vi "FVIR_LDO_Alicat_GasMeter.vi"(8 "error in":errorcluster, 11 "Message Queues":T1) -> (0 "error out":errorcluster)   [LabVIEW 2020]
uses:
  Message Queue/All Message Queues.ctl
  Message Queue/Message Cluster.ctl
  Modbus/Modbus Gas Meter Data.ctl
  Drivers/Alicat LabVIEW Drivers 2v1/Sub-VIs/Data Cluster.ctl
  Drivers/Alicat LabVIEW Drivers 2v1/Sub-VIs/Units of Measure.ctl
  Message Queue/Enqueue Message (Single).vi
  Message Queue/Message Queue.lvlib
panel:
  out "Numeric":i32
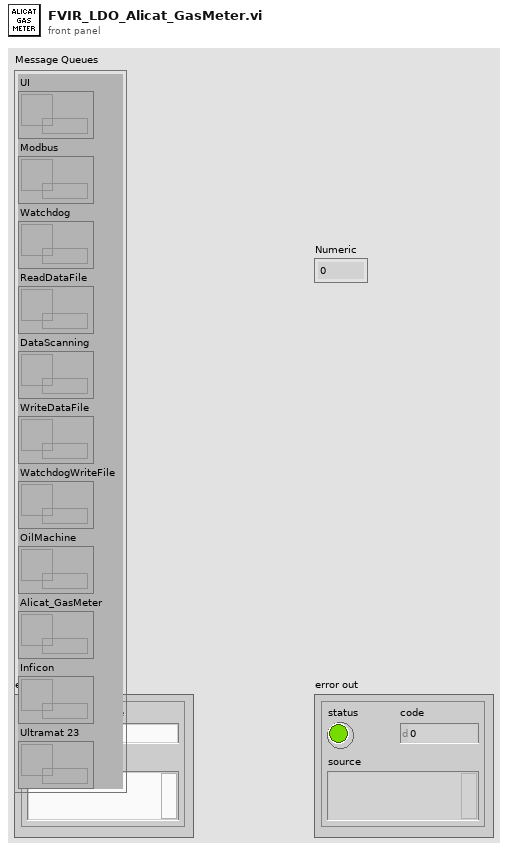
[diagram p1: front panel]
types:
  T1 = typedef "Message Queue.lvlib/All Message Queues.ctl" = cluster{"UI":refnum<queue>, "Modbus":refnum<queue>, "Watchdog":refnum<queue>, "ReadDataFile":refnum<queue>, "DataScanning":refnum<queue>, "WriteDataFile":refnum<queue>, "WatchdogWriteFile":refnum<queue>, "OilMachine":refnum<queue>, "Alicat_GasMeter":refnum<queue>, "Inficon":refnum<queue>, "Ultramat 23":refnum<queue>}
  T2 = cluster{"Absolute Press.":bool, "Gauge/Diff. Press.":bool, "Barometric Press.":bool, "Temperature":bool, "Volumetric":bool, "Mass Flow":bool, "Setpoint":bool, "Valve Drive":bool, "Totalizer":bool, "Tot. Timer [s]":bool, "Tot. Avg. Flow":bool, "Tot. Peak Flow":bool, "Gas Selected":bool, "Log Data":bool}
  T3 = typedef "Modbus Gas Meter Data.ctl" = cluster{"Data Cluster":T4, "Units of Measure Input":T5, "Header Array":string[]}
  T4 = typedef "Data Cluster.ctl" = cluster{"Absolute Pressure":dbl, "Gauge/Diff. Pressure":dbl, "Barometric Pressure":dbl, "Temperature":dbl, "Volumetric Flow":dbl, "Mass Flow":dbl, "Setpoint":dbl, "Valve Drive":dbl, "Totalizer":dbl, "[hr]":dbl, "[min]":dbl, "[sec]":dbl, "Totalizer Average Flow":dbl, "Totalizer Peak Flow":dbl, "Gas selected":string}
  T5 = typedef "Units of Measure.ctl" = cluster{"Abs. Pressure":string, "Gauge/Diff. Press.":string, "Barometric Press.":string, "Temperature":string, "Volume":string, "Mass":string, "Setpoint":string, "Valve Drive":string, "Totalizer":string, "Tot. Timer":string, "Tot. Avg. Flow":string, "Tot. Peak Flow":string}
  T6 = typedef "Data Frame.ctl" = cluster{"Absolute Pressure":bool, "Gauge/Diff. Pressure":bool, "Barometric Pressure":bool, "Temperature":bool, "Volumetric":bool, "Mass":bool, "Setpoint":bool, "Valve Drive":bool, "Totalizer":bool, "Totalizer Timer":bool, "Totalizer Average Flow":bool, "Totalizer Peak Flow":bool, "Gas Selected":bool, "Tot. Timer Format":u16}
  T7 = typedef "FMA1600A Units String.ctl" = cluster{"Software Rev":string, "Model Number":string, "Manufacturer Info":string, "Software Sub-Rev":string, "Board Rev":string, "Units of Measure Input":T5}
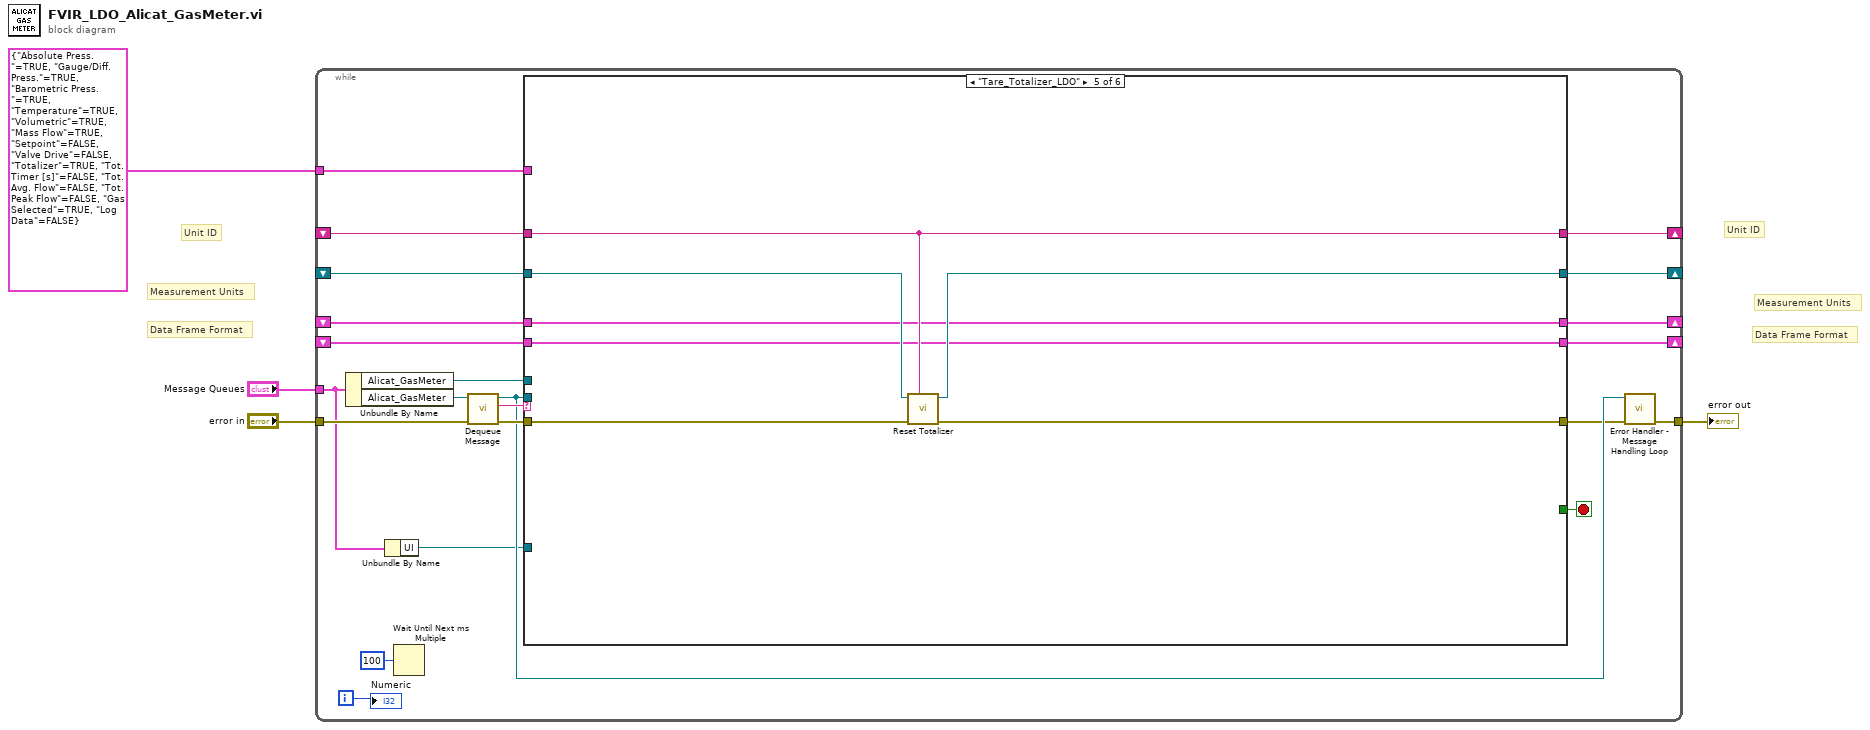
[diagram p0: block diagram]
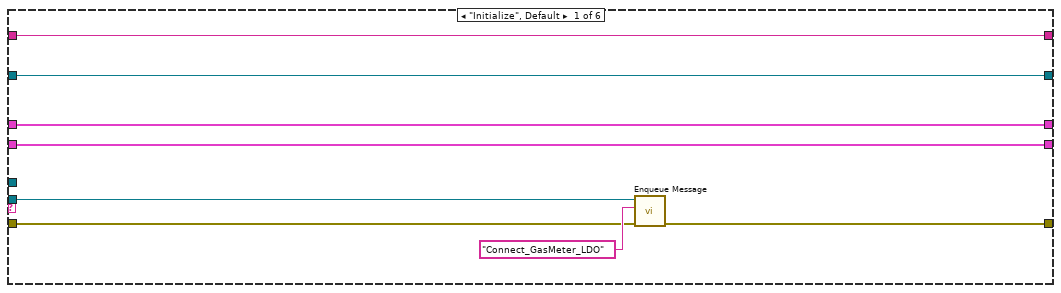
[diagram p2: hidden frame]
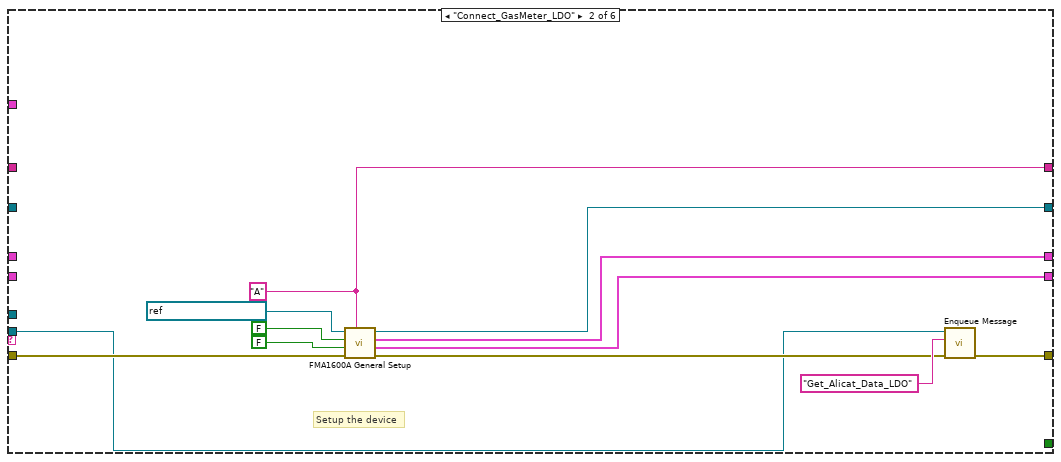
[diagram p3: hidden frame]
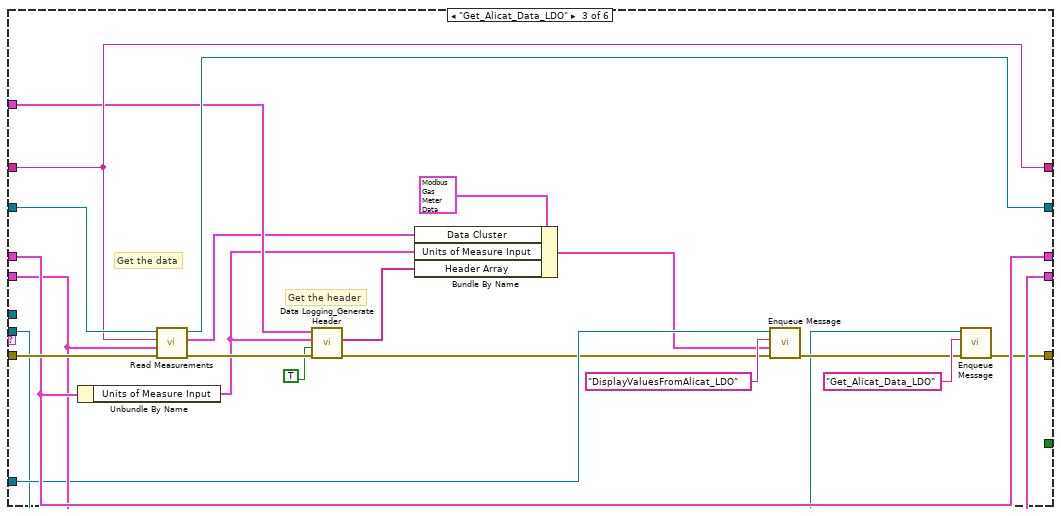
[diagram p4: hidden frame]
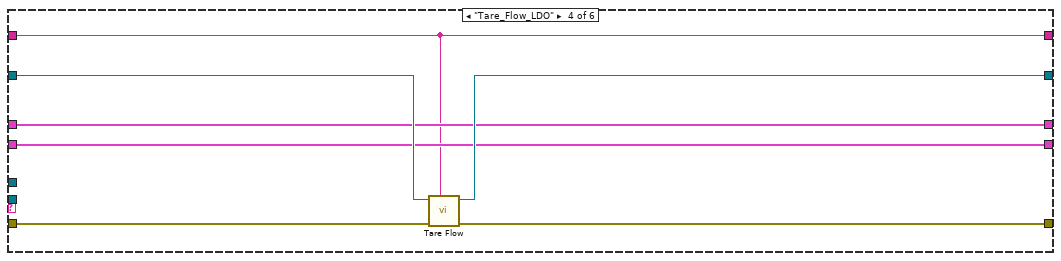
[diagram p5: hidden frame]
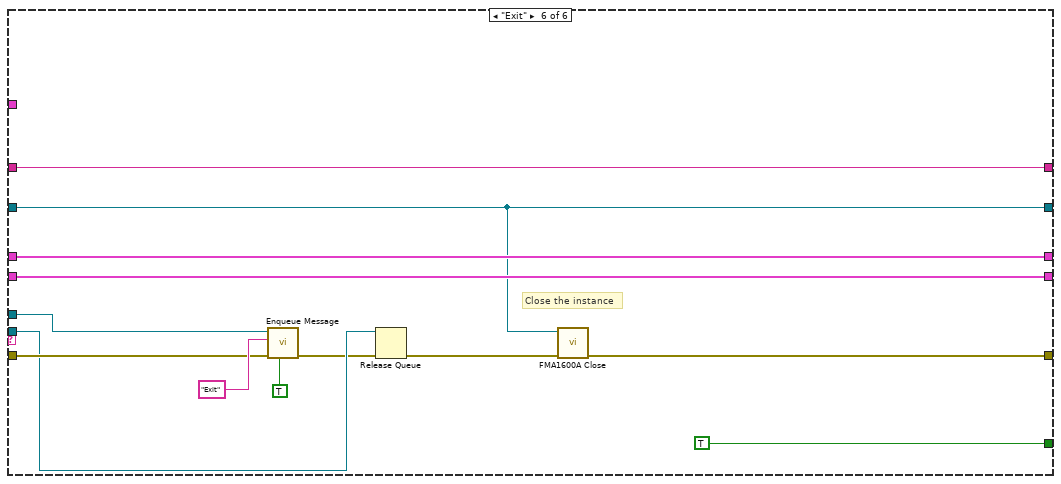
[diagram p6: hidden frame]
diagram:
  # "Unit ID"
  # "Data Frame Format"
  # "Measurement Units"
  # "Unit ID"
  # "Data Frame Format"
  # "Measurement Units"
  n1 = while {
    tunnel: "Message Queues" -> [w6]
    tunnel: "error in" -> [w25]
    tunnel: [w19] -> w2
    shift-right: [w17] -> _
    shift-left: _ -> [w16]
    shift-right: [w13] -> _
    shift-left: _ -> [w10]
    shift-right: [w12] -> _
    shift-left: _ -> [w11]
    shift-right: [w9] -> _
    shift-left: _ -> [w8]
    tunnel: T2 {"Absolute Press."=TRUE, "Gauge/Diff. Press."=TRUE, "Barometric Press."=TRUE, "Temperature"=TRUE, "Volumetric"=TRUE, "Mass Flow"=TRUE, "Setpoint"=FALSE, "Valve Drive"=FALSE, "Totalizer"=TRUE, "Tot. Timer [s]"=FALSE, "Tot. Avg. Flow"=FALSE, "Tot. Peak Flow"=FALSE, "Gas Selected"=TRUE, "Log Data"=FALSE} ("Data Logging Options") -> [w7]
    i -> [w14]
    stop <- w22 stop-if-true
    n2 = Unbundle By Name(w6) -> ("Alicat_GasMeter"=w21:refnum<queue>, "Alicat_GasMeter"=w26:refnum<queue>)
    n3 = Unbundle By Name(w6) -> ("UI"=w5:refnum<queue>)
    n4 = Wait Until Next ms Multiple(millisecond multiple=u32 100) -> ()  [unwired: 1 out]
    n5 = call "Dequeue Message.vi"("error in (no error)"=w25, "Message Queue"=w26) -> ("error out"=w23:errorcluster, "Message"=w24:string, "dup Message Queue"=w20:refnum<queue>)  [unwired: 6 in, 1 out]
    n6 = case shown="\"Tare_Totalizer_LDO\"" w24 {
      tunnel: w23 -> [w29 w43 w64 w74 w81 w90]
      tunnel: [w28 w36 w54 w73 w80 w86] -> w18
      tunnel: [_ _ _ _ _ TRUE] -> w22
      tunnel: w21 -> [_ _ _ _ _ w91]
      tunnel: w20 -> [w27 w35 w53 _ _ w89]
      tunnel: [w34 w42 w65 w71 w77 w82] -> w17
      tunnel: w16 -> [w34 _ w63 w72 w79 w82]
      tunnel: [w32 w41 w61 w70 w76 w84] -> w13
      tunnel: [w31 w40 w60 w69 w75 w83] -> w12
      tunnel: w11 -> [w31 _ w60 w69 w75 w83]
      tunnel: w10 -> [w32 _ w61 w70 w76 w84]
      tunnel: [w33 w39 w62 w68 w78 w85] -> w9
      tunnel: w8 -> [w33 _ w62 w68 w78 w85]
      tunnel: w7 -> [_ _ w59 _ _ _]
      tunnel: w5 -> [_ _ w57 _ _ _]
      frame "Initialize", Default {
        n7 = call-poly "Enqueue Message.vi"("error in (no error)"=w29, "Message"="Connect_GasMeter_LDO", "Message Queue"=w27) -> ("error out"=w28:errorcluster)  [unwired: 7 in, 1 out]
      }
      frame "Connect_GasMeter_LDO" {
        w39 = "A" ("Unit ID")
        # "Setup the device"
        n8 = call "FMA1600A General Setup.vi"("Unit ID"=w39, "error in (no error)"=w43, "Select Gas?"=FALSE, "Set STP Register"=FALSE, "VISA Refnum in"=refnum<visa-resource-name> "ALICAT_100SLPM") -> ("error out"=w37:errorcluster, "Data Frame Format"=w40:T6, "Measurement Units"=w41:T7, "VISA Refnum out"=w42:refnum<visa-resource-name>)  [unwired: 3 in]
        n9 = call-poly "Enqueue Message.vi"("error in (no error)"=w37, "Message"="Get_Alicat_Data_LDO", "Message Queue"=w35) -> ("error out"=w36:errorcluster)  [unwired: 7 in, 1 out]
      }
      frame "Get_Alicat_Data_LDO" {
        # "Get the header"
        # "Get the data"
        n10 = Unbundle By Name(w61) -> ("Units of Measure Input"=w49:T5)
        n11 = call "Read Measurements.vi"("error in"=w64, "Data Frame Format In"=w60, "Unit ID (A)"=w62, "VISA Session In"=w63) -> ("error out"=w67:errorcluster, "Data Cluster"=w50:T4, "VISA Session Out"=w65:refnum<visa-resource-name>)  [unwired: 5 out]
        n12 = call "Data Logging_Generate Header.vi"("error in"=w67, "Include Units\nin Header (F)"=TRUE ("Include Units\nin Header (default is F)"), "Units of Measure Input"=w49, "Data Logging Options"=w59) -> ("error out"=w52:errorcluster, "Header Array"=w48:string[])  [unwired: 5 in, 1 out]
        n13 = Bundle By Name(cluster=T3 {"Data Cluster"={"Absolute Pressure"=0.0, "Gauge/Diff. Pressure"=0.0, "Barometric Pressure"=0.0, "Temperature"=0.0, "Volumetric Flow"=0.0, "Mass Flow"=0.0, "Setpoint"=0.0, "Valve Drive"=0.0, "Totalizer"=0.0, "[hr]"=0.0, "[min]"=0.0, "[sec]"=0.0, "Totalizer Average Flow"=0.0, "Totalizer Peak Flow"=0.0, "Gas selected"=""}, "Units of Measure Input"={"Abs. Pressure"="", "Gauge/Diff. Press."="", "Barometric Press."="", "Temperature"="", "Volume"="", "Mass"="", "Setpoint"="", "Valve Drive"="", "Totalizer"="", "Tot. Timer"="", "Tot. Avg. Flow"="", "Tot. Peak Flow"=""}, "Header Array"=[]} ("Gas Data"), "Data Cluster"=w50, "Units of Measure Input"=w49, "Header Array"=w48) -> (w47:T3)
        n14 = call-poly "Enqueue Message.vi"("error in (no error)"=w52, "Message Data"=w47, "Message"="DisplayValuesFromAlicat_LDO", "Message Queue"=w57) -> ("error out"=w55:errorcluster)  [unwired: 6 in, 1 out]
        n15 = call-poly "Enqueue Message.vi"("error in (no error)"=w55, "Message"="Get_Alicat_Data_LDO", "Message Queue"=w53) -> ("error out"=w54:errorcluster)  [unwired: 7 in, 1 out]
      }
      frame "Tare_Flow_LDO" {
        n16 = call "Tare Flow.vi"("Unit ID (A)"=w68, "error in"=w74, "VISA Session In"=w72) -> ("error out"=w73:errorcluster, "VISA Session Out"=w71:refnum<visa-resource-name>)  [unwired: 7 in]
      }
      frame "Tare_Totalizer_LDO" {
        n17 = call "Reset Totalizer.vi"("Unit ID (A)"=w78, "error in"=w81, "VISA Session In"=w79) -> ("error out"=w80:errorcluster, "VISA Session Out"=w77:refnum<visa-resource-name>)  [unwired: 6 in, 1 out]
      }
      frame "Exit" {
        # "Close the instance"
        n18 = call-poly "Enqueue Message.vi"("Priority Message? (F)"=TRUE, "error in (no error)"=w90, "Message"="Exit", "Message Queue"=w91) -> ("error out"=w88:errorcluster)  [unwired: 6 in, 1 out]
        n19 = Release Queue(queue=w89, error in (no error)=w88) -> (error out=w87:errorcluster)  [unwired: 1 in, 2 out]
        n20 = call "FMA1600A Close.vi"("error in (no error)"=w87, "VISA Refnum in"=w82) -> ("error out"=w86:errorcluster)  [unwired: 9 in]
      }
    }
    n21 = call "Error Handler - Message Handling Loop.vi"("error in (no error)"=w18, "Message Queue"=w20) -> ("dup error in"=w19:errorcluster)  [unwired: 8 in, 1 out]
    "Numeric" <- w14
  }
  "error out" <- w2
